vi "axex_write_cells.vi"(8 "error in":errorcluster, 9 "cell array":string[][](array[string]), 10 "top left cell":T1, 11 "AX Excel instance in":T2) -> (0 "error out":errorcluster, 3 "AX Excel instance out":T2)   [LabVIEW 2020, in "AX Excel.lvlib"]
doc: "Call this to write array of cells. Array coordinates are given by top-left cell coordinates. The coordinates may be given as [column,row] index or cell name such as A1, AB66, ... with priority of cell name."
uses:
  AX Excel.lvlib
  axex_instance.ctl
  axex_cell_xy.ctl
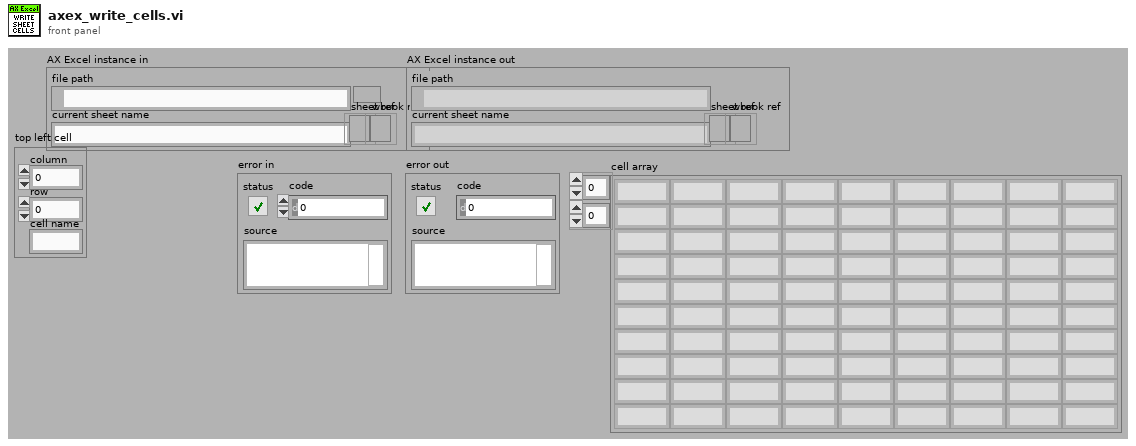
[diagram p1: front panel]
types:
  T1 = typedef "AX Excel.lvlib/axex_cell_xy.ctl" = cluster{"column":i32, "row":i32, "cell name":string}
  T2 = typedef "AX Excel.lvlib/axex_instance.ctl" = cluster{"file path":path, "current sheet name":string, "sheet ref":refnum<k7>, "wbook ref":refnum<k7>}
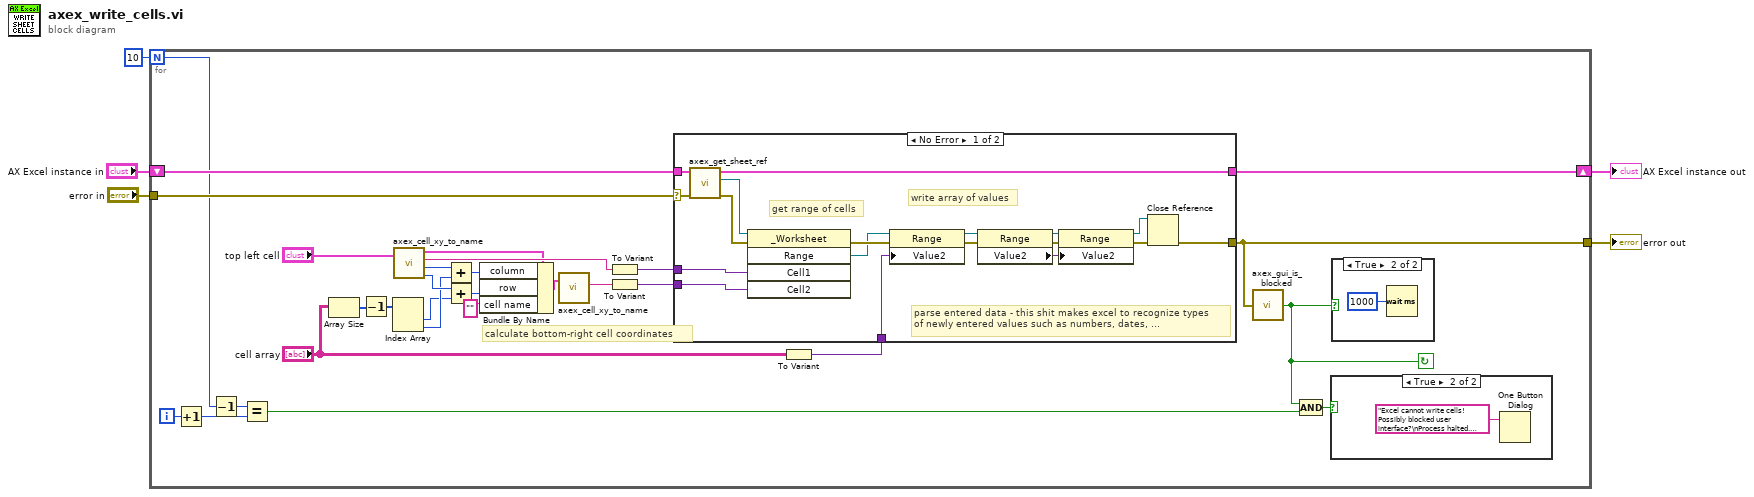
[diagram p0: block diagram]
diagram:
  n1 = for {
    N: 10 -> [w12]
    tunnel: "error in" -> [w14]
    tunnel: [w13] -> w2
    shift-right: [w33] -> w4
    shift-left: "AX Excel instance in" -> [w34]
    i -> [w11]
    stop <- w7 continue-if-true
    # "calculate bottom-right cell coordinates"
    n2 = Increment(x=w11) -> (x+1=w10:i32)
    n3 = Decrement(x=w12) -> (x-1=w6:i32)
    n4 = Equal?(x=w6, y=w10) -> (x = y?=w9:bool)
    n5 = Array Size(array="cell array") -> (size(s)=w27:i32[])
    n6 = Decrement(x=w27) -> (x-1=w24:i32[])
    n7 = Index Array(array=w24) -> (element #1=w16:i32, element #2=w17:i32)  [unwired: 2 in]
    n8 = call "axex_cell_xy_to_name.vi"("cell xy in"="top left cell") -> ("cell xy out"=w25:T1, "cell name"=w28:string, "column"=w22:i32, "row"=w19:i32)  [unwired: 1 in]
    n9 = Add(x=w22, y=w17) -> (x+y=w21:i32)
    n10 = Add(x=w19, y=w16) -> (x+y=w20:i32)
    n11 = Bundle By Name(cluster=w25, "column"=w21, "row"=w20, "cell name"="") -> (w26:T1)
    n12 = call "axex_cell_xy_to_name.vi"("cell xy in"=w26) -> ("cell name"=w29:string)  [unwired: 1 in, 3 out]
    n13 = To Variant(anything=w28) -> (Variant=w32:variant)
    n14 = To Variant(anything=w29) -> (Variant=w31:variant)
    n15 = To Variant(anything="cell array") -> (Variant=w15:variant)
    n16 = case shown="No Error" w14 {
      selector: w14 -> [w37 w56]
      tunnel: w34 -> [w54 w55]
      tunnel: [w53 w55] -> w33
      tunnel: w32 -> [w51 _]
      tunnel: w31 -> [w50 _]
      tunnel: [w48 w56] -> w13
      tunnel: w15 -> [w45 _]
      frame No Error {
        # "parse entered data - this shit makes excel to recognize types\nof newly entered values such as numbers, dates, ..."
        # "write array of values"
        # "get range of cells"
        n17 = call "axex_get_sheet_ref.vi"("error in"=w37, "AX Excel instance in"=w54) -> ("error out"=w49:errorcluster, "sheet ref out"=w52:refnum<k7>, "AX Excel instance out"=w53:T2)  [unwired: 6 in, 1 out]
        n18 = invoke class="_Worksheet" method="Range"(reference=w52, error in=w49, "Cell1"=w51, "Cell2"=w50) -> (error out=w47:errorcluster, "Range"=w46:refnum<k7>)  [unwired: 1 in, 3 out]
        n19 = property class="Range"(reference=w46, error in=w47, "Value2"=w45) -> (reference out=w44:refnum<k7>, error out=w43:errorcluster)
        n20 = property class="Range"(reference=w44, error in=w43) -> (reference out=w40:refnum<k7>, error out=w41:errorcluster, "Value2"=w42:variant)
        n21 = property class="Range"(reference=w40, error in=w41, "Value2"=w42) -> (reference out=w38:refnum<k7>, error out=w39:errorcluster)
        n22 = Close Reference(reference=w38, error in (no error)=w39) -> (error out=w48:errorcluster)
      }
      frame Error {
      }
    }
    n23 = call "axex_gui_is_blocked.vi"("error in"=w13) -> ("gui blocked?"=w7:bool)
    n24 = Compound Arithmetic op=AND(w7, w9) -> (w8:bool)
    n25 = case shown="True" w8 {
      frame False {
      }
      frame True {
        n26 = One Button Dialog(message="Excel cannot write cells! Possibly blocked user interface?\nProcess halted. Press ok to retry.") -> ()  [unwired: 1 in, 1 out]
      }
    }
    n27 = case shown="True" w7 {
      frame False {
      }
      frame True {
        n28 = Wait (ms)(milliseconds to wait=u32 1000) -> ()  [unwired: 1 out]
      }
    }
  }
  "error out" <- w2
  "AX Excel instance out" <- w4
